vi "Add State.vi"(8 "error in":errorcluster, 10 "State":string, 11 "History in":refnum<class "History.lvclass">) -> (0 "error out":errorcluster, 3 "History out":refnum<class "History.lvclass">)   [LabVIEW 2020, in "lv_icon.lvlib" / "History.lvlib" / "History.lvclass"]
doc: "Adds a state to the undo stack.\n\nThis process clears the available redo states."
uses:
  History.lvclass
  History.lvclass/History.ctl
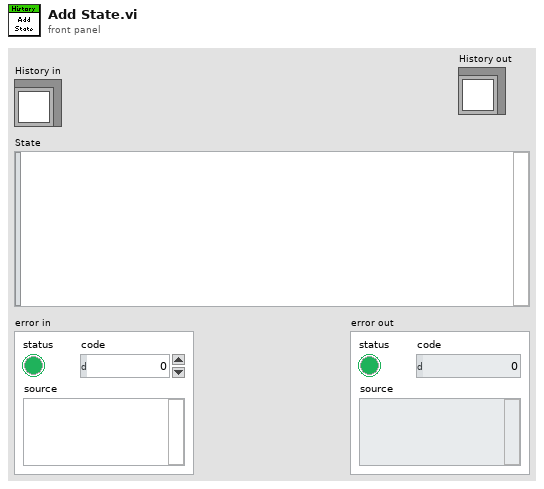
[diagram p1: front panel]
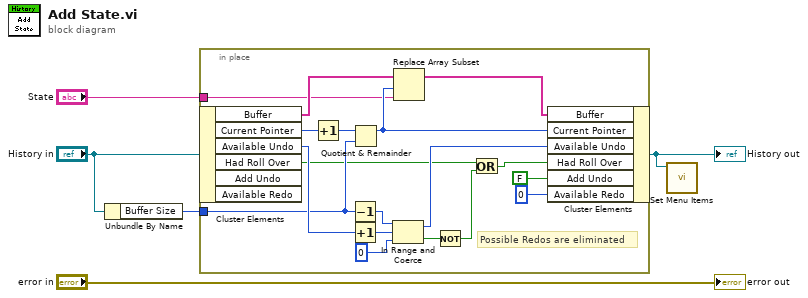
[diagram p0: block diagram]
diagram:
  n1 = Unbundle By Name("History in") -> ("Buffer Size"=w3:i32)
  n2 = in-place {
    in-place-border: w3 -> [w15]
    in-place-border: "State" -> [w11]
    # "Possible Redos are eliminated"
    n3 = in-place-cluster #1("History in") -> ("Buffer"=w14:string[], "Current Pointer"=w21:i32, "Available Undo"=w23:i32, "Had Roll Over"=w9:bool)  [unwired: 2 out]
    n4 = Increment(x=w21) -> (x+1=w22:i32)
    n5 = Decrement(x=w15) -> (x-1=w16:i32)
    n6 = Increment(x=w23) -> (x+1=w19:i32)
    n7 = Quotient & Remainder(x=w22, y=w15) -> (x-y*floor(x/y)=w12:i32)  [unwired: 1 out]
    n8 = In Range and Coerce(upper limit=w16, x=w19, lower limit=0) -> (coerced(x)=w10:i32, In Range?=w18:bool)
    n9 = Replace Array Subset(array=w14, new element=w11, index=w12) -> (w13:string[])
    n10 = Not(x=w18) -> (.not. x?=w17:bool)
    n11 = Or(x=w9, y=w17) -> (x .or. y?=w8:bool)
    n12 = in-place-cluster #1("Buffer"=w13, "Current Pointer"=w12, "Available Undo"=w10, "Had Roll Over"=w8, "Add Undo"=FALSE, "Available Redo"=0) -> (w1:refnum<class "History.lvclass">)
  }
  "History out" <- w1
  n13 = call "Set Menu Items.vi"("History"=w1) -> ()  [unwired: 11 in]
  "error out" <- "error in"
